vi "Set Server gRPC UEs.vi"(10 "Server gRPC UEs":T1, 11 "OOP Server in":refnum<class "HVC9.lvclass">) -> (3 "OOP Server out":refnum<class "HVC9.lvclass">)   [LabVIEW 2019, in "HVC9.lvlib" / "HVC9.lvclass"]
uses:
  HVC9.lvclass
  typeDefs/Server gRPC UEs.ctl
  gRPC lvSupport/Server API/typeDefs/gRPCId Cluster.ctl
  gRPC lvSupport/Server API/typeDefs/grpcId.ctl
  HVC9.lvclass/HVC9.ctl
  gRPC lvSupport/gprc-lvsupport.lvlib
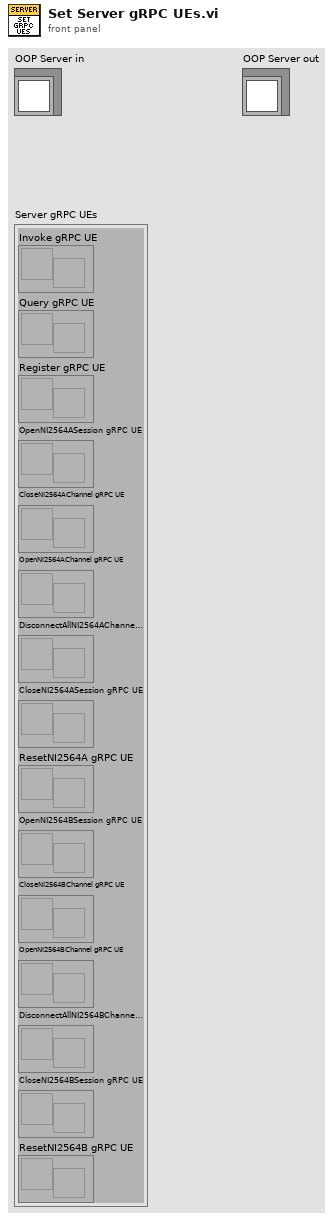
[diagram p1: front panel]
types:
  T1 = typedef "HVC9.lvlib/HVC9.lvclass/Server gRPC UEs.ctl" = cluster{"Invoke gRPC UE":refnum<user-event>, "Query gRPC UE":refnum<user-event>, "Register gRPC UE":refnum<user-event>, "OpenNI2564ASession gRPC UE":refnum<user-event>, "CloseNI2564AChannel gRPC UE":refnum<user-event>, "OpenNI2564AChannel gRPC UE":refnum<user-event>, "DisconnectAllNI2564AChannels gRPC UE":refnum<user-event>, "CloseNI2564ASession gRPC UE":refnum<user-event>, "ResetNI2564A gRPC UE":refnum<user-event>, "OpenNI2564BSession gRPC UE":refnum<user-event>, "CloseNI2564BChannel gRPC UE":refnum<user-event>, "OpenNI2564BChannel gRPC UE":refnum<user-event>, "DisconnectAllNI2564BChannels gRPC UE":refnum<user-event>, "CloseNI2564BSession gRPC UE":refnum<user-event>, "ResetNI2564B gRPC UE":refnum<user-event>}
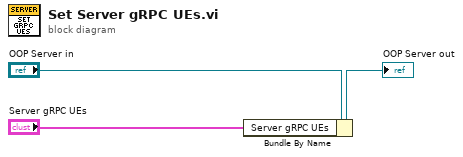
[diagram p0: block diagram]
diagram:
  n1 = Bundle By Name(cluster="OOP Server in", "Server gRPC UEs"="Server gRPC UEs") -> (→"OOP Server out":refnum<class "HVC9.lvclass">)
